vi "Get Shift.vi"(8 "error in (no error)":errorcluster, 10 "Time Stamp Out":timestamp[](array[timestamp])) -> (0 "error out":errorcluster, 2 "Shift":i32)   [LabVIEW 2017]
panel:
  out "double precision float":dbl format="%#_13g"
  in  "Shift Time Details":T1 {"3End" format="%<%H:%M:%S\n%x>T"; "2End" format="%<%H:%M:%S\n%x>T"; "3Start" format="%<%H:%M:%S\n%x>T"; "2Start" format="%<%H:%M:%S\n%x>T"; "1End" format="%<%H:%M:%S\n%x>T"; "1Start" format="%<%H:%M:%S\n%x>T"}
  # "Start Time"
  # "End Time"
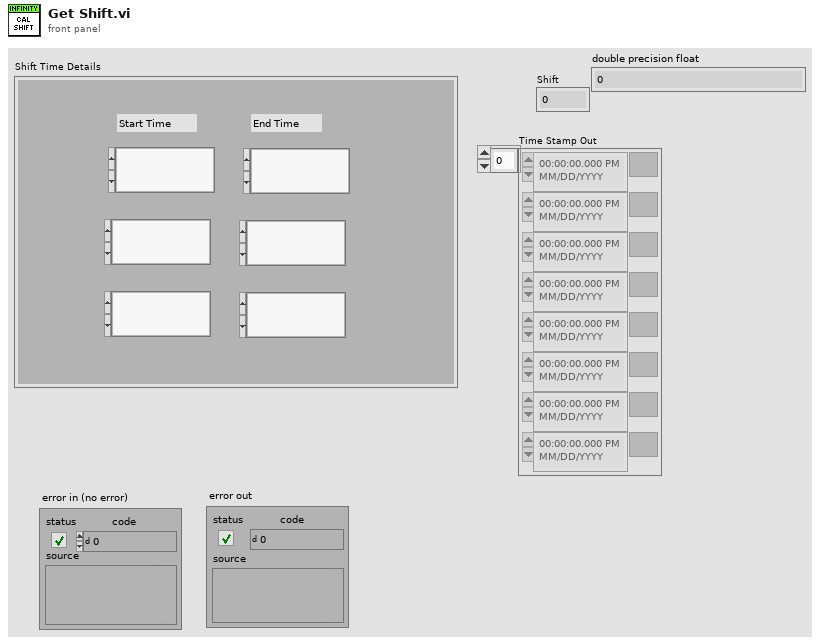
[diagram p1: front panel]
types:
  T1 = cluster{"1Start":timestamp, "1End":timestamp, "2Start":timestamp, "3Start":timestamp, "2End":timestamp, "3End":timestamp}
  T2 = typedef "LVDateTimeRec.ctl" = cluster{"fractional second":dbl, "second":i32, "minute":i32, "hour":i32, "day of month":i32, "month":i32, "year":i32, "day of week":i32, "day of year":i32, "DST":i32}
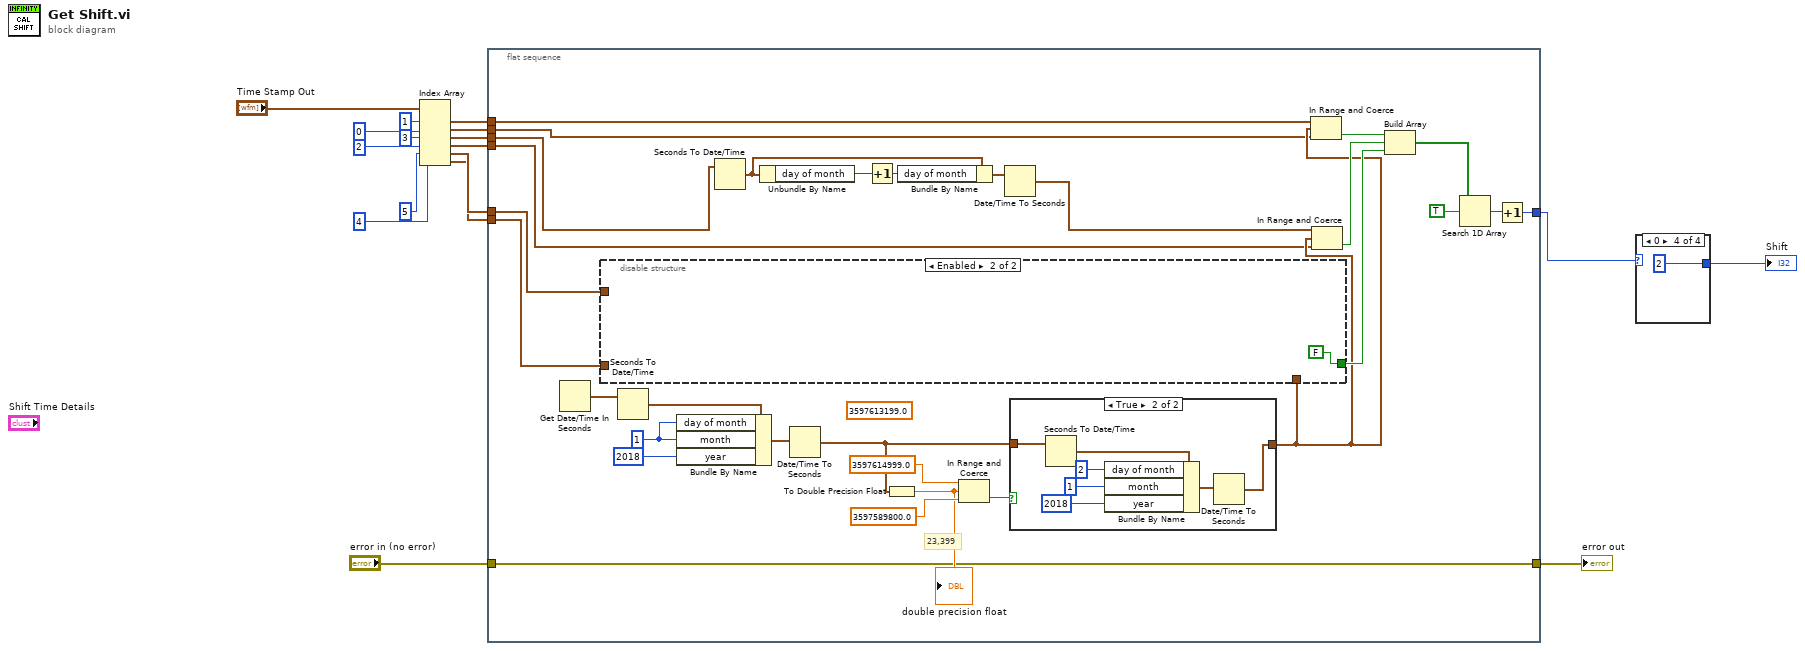
[diagram p0: block diagram]
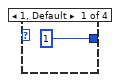
[diagram p2: hidden frame]
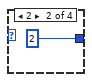
[diagram p3: hidden frame]
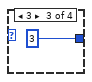
[diagram p4: hidden frame]
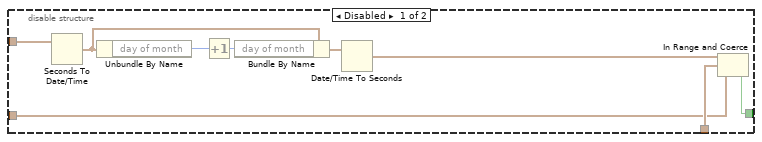
[diagram p5: hidden frame]
diagram:
  n1 = Index Array(array="Time Stamp Out", index #1=1 ("index"), index #2=0 ("index"), index #3=3 ("index"), index #4=2 ("index"), index #5=5 ("index"), index #6=4 ("index")) -> (element #1=w12:timestamp, element #2=w11:timestamp, element #3=w8:timestamp, element #4=w7:timestamp, element #5=w4:timestamp, element #6=w3:timestamp)
  n2 = flat-sequence {
    tunnel: [w41] -> w2
    tunnel: "error in (no error)" -> [w30]
    tunnel: [w30] -> w16
    tunnel: w12 -> [w29]
    tunnel: w11 -> [w28]
    tunnel: w8 -> [w19]
    tunnel: w7 -> [w27]
    tunnel: w4 -> [w26]
    tunnel: w3 -> [w25]
    frame #0 {
      (unwired) 3597613199.0 ("double precision float 2")
      w34 = 1 ("day of month")
      # "23,399"
      n3 = Get Date/Time In Seconds() -> (seconds since 1Jan1904=w24:timestamp)
      n4 = Seconds To Date/Time(time stamp (now)=w24) -> (date time rec=w38:T2)  [unwired: 1 in]
      n5 = Bundle By Name(cluster=w38, "day of month"=w34, "month"=w34, "year"=2018) -> (w40:T2)
      n6 = Seconds To Date/Time(time stamp (now)=w19) -> (date time rec=w22:T2)  [unwired: 1 in]
      n7 = Unbundle By Name(w22) -> ("day of month"=w20:i32)
      n8 = Date/Time To Seconds(2:w40) -> (0:w32:timestamp)  [unwired: 1 in]
      n9 = Increment(x=w20) -> (x+1=w21:i32)
      n10 = To Double Precision Float(number=w32) -> (double precision float=w35:dbl)
      "double precision float" <- w35
      n11 = Bundle By Name(cluster=w22, "day of month"=w21) -> (w23:T2)
      n12 = In Range and Coerce(upper limit=3597614999.0 ("double precision float 2"), x=w35, lower limit=3597589800.0 ("double precision float")) -> (In Range?=w33:bool)  [unwired: 1 out]
      n13 = Date/Time To Seconds(2:w23) -> (0:w18:timestamp)  [unwired: 1 in]
      n14 = case shown="True" w33 {
        tunnel: w32 -> [w58 w61]
        tunnel: [w58 w60] -> w31
        frame False {
        }
        frame True {
          n15 = Seconds To Date/Time(time stamp (now)=w61) -> (date time rec=w63:T2)  [unwired: 1 in]
          n16 = Bundle By Name(cluster=w63, "day of month"=2, "month"=1 ("day of month"), "year"=2018) -> (w65:T2)
          n17 = Date/Time To Seconds(2:w65) -> (0:w60:timestamp)  [unwired: 1 in]
        }
      }
      n18 = disable-structure shown="Enabled" {
        disable-tunnel: [w55 FALSE] -> w45
        disable-tunnel: w31 -> [w54 _]
        disable-tunnel: w26 -> [w53 _]
        disable-tunnel: w25 -> [w52 _]
        frame Disabled {
          n19 = Seconds To Date/Time(time stamp (now)=w53) -> (date time rec=w50:T2)  [unwired: 1 in]
          n20 = Unbundle By Name(w50) -> ("day of month"=w48:i32)
          n21 = Increment(x=w48) -> (x+1=w49:i32)
          n22 = Bundle By Name(cluster=w50, "day of month"=w49) -> (w51:T2)
          n23 = Date/Time To Seconds(2:w51) -> (0:w56:timestamp)  [unwired: 1 in]
          n24 = In Range and Coerce(upper limit=w56, x=w54, lower limit=w52) -> (In Range?=w55:bool)  [unwired: 1 out]
        }
        frame Enabled {
        }
      }
      n25 = In Range and Coerce(upper limit=w29, x=w31, lower limit=w28) -> (In Range?=w47:bool)  [unwired: 1 out]
      n26 = In Range and Coerce(upper limit=w18, x=w31, lower limit=w27) -> (In Range?=w46:bool)  [unwired: 1 out]
      n27 = Build Array(w47, w46, w45) -> (w44:bool[])
      n28 = Search 1D Array(1D array=w44, element=TRUE) -> (index of element=w42:i32)  [unwired: 1 in]
      n29 = Increment(x=w42) -> (x+1=w41:i32)
    }
  }
  n30 = case shown="0" w2 {
    tunnel: [1 2 3 2] -> w1
    frame 1, Default {
    }
    frame 2 {
    }
    frame 3 {
    }
    frame 0 {
    }
  }
  "Shift" <- w1
  "error out" <- w16
